vi "Or77200_DoXSteps.vi"(6 "MoveRef":refnum<vi>, 7 "Stop Ref":refnum<vi>, 8 "error In":errorcluster caption="error out", 9 "Dir (Dec:F)":bool caption="Dir", 10 "Steps":u32, 11 "Port":refnum<visa-resource-name>) -> (0 "sortie d'erreur":errorcluster, 2 "sortie 1":i32, 3 "Port Out":refnum<visa-resource-name>)   [LabVIEW 2019]
uses:
  <userlib>/GenProg/WritebyWeakRefBool.vi
  <userlib>/GenProg/ReadbyWeakRefBool.vi
panel:
  out "Moving":bool
  in  "Stop":bool
  out "Response":string
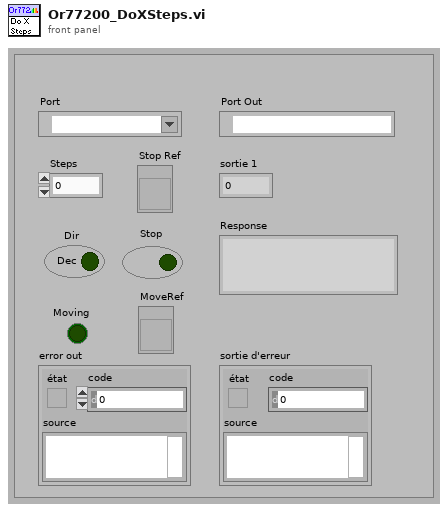
[diagram p1: front panel]
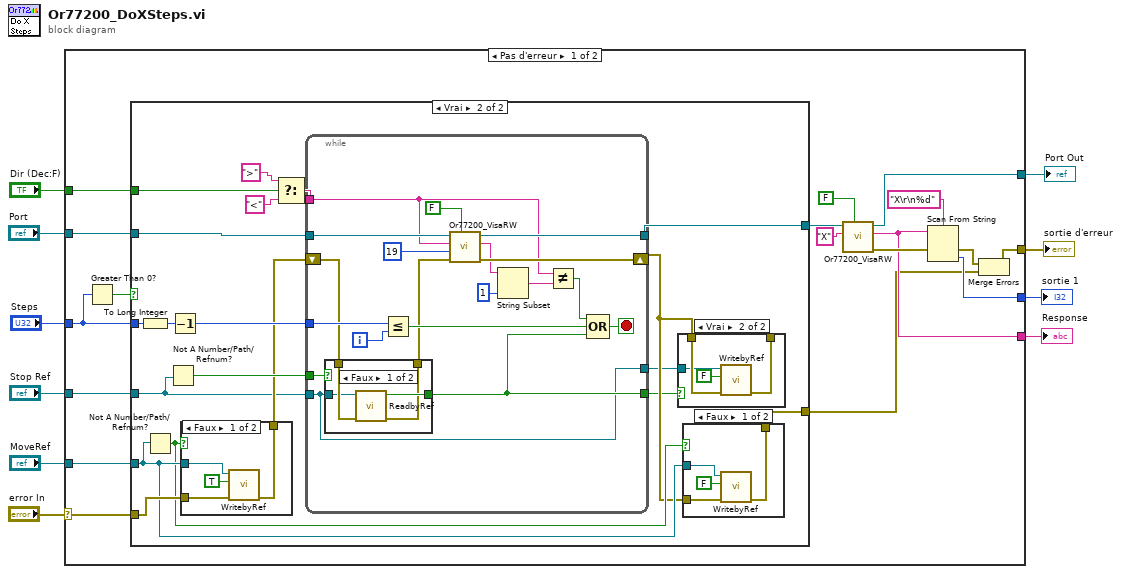
[diagram p0: block diagram]
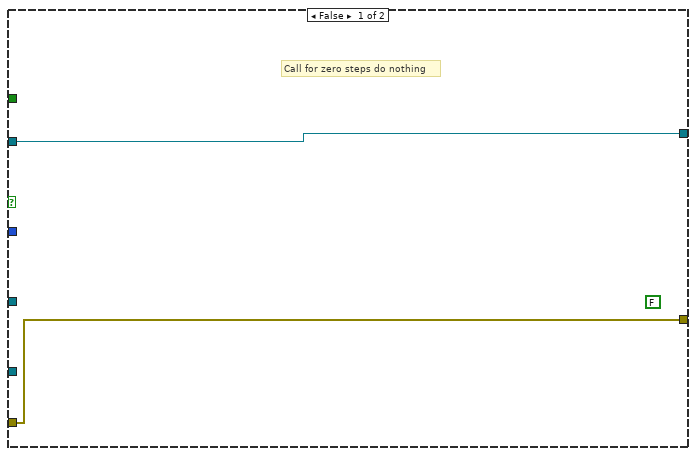
[diagram p2: hidden frame]
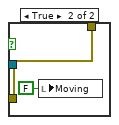
[diagram p4: hidden frame]
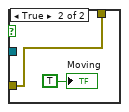
[diagram p5: hidden frame]
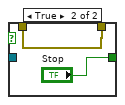
[diagram p6: hidden frame]
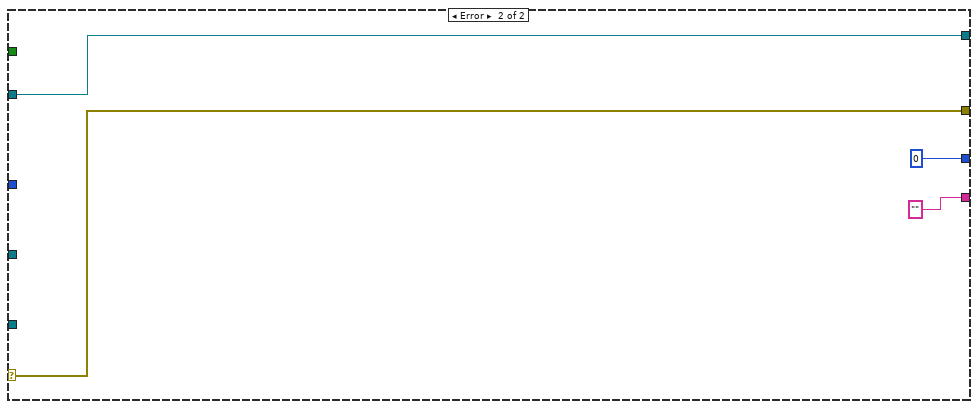
[diagram p7: hidden frame]
diagram:
  n1 = case shown="Pas d'erreur" "error In" {
    selector: "error In" -> [w18 w94]
    tunnel: "Port" -> [w28 w95]
    tunnel: "Dir (Dec:F)" -> [w27 _]
    tunnel: "Steps" -> [w16 _]
    tunnel: [w23 0] -> w7
    tunnel: [w14 w94] -> w6
    tunnel: [w21 w95] -> w5
    tunnel: "Stop Ref" -> [w19 _]
    tunnel: [w20 "" ("Response")] -> w3
    tunnel: "MoveRef" -> [w11 _]
    frame No Error {
      n2 = Greater Than 0?(x=w16) -> (x > 0?=w17:bool)
      n3 = case shown="Vrai" w17 {
        tunnel: w28 -> [w29 w49]
        tunnel: w27 -> [_ w48]
        tunnel: w16 -> [_ w47]
        tunnel: [w30 w37] -> w13
        tunnel: [w29 w45] -> w25
        tunnel: w19 -> [_ w34]
        tunnel: w18 -> [w30 w39]
        tunnel: w11 -> [_ w36]
        frame False {
          (unwired) FALSE ("Stop")
          # "Call for zero steps do nothing"
        }
        frame True {
          n4 = To Long Integer(number=w47) -> (32bit integer=w41:i32)
          n5 = Not A Number/Path/Refnum?(number/path/refnum=w36) -> (NaN/Path/Refnum?=w35:bool)
          n6 = Not A Number/Path/Refnum?(number/path/refnum=w34) -> (NaN/Path/Refnum?=w42:bool)
          n7 = Decrement(x=w41) -> (x-1=w46:i32)
          n8 = case shown="Faux" w35 {
            tunnel: [w64 w66] -> w38
            tunnel: w36 -> [w63 _]
            tunnel: w39 -> [w62 w66]
            frame False {
              n9 = call-poly <userlib>:"WritebyRef.vi"("error in"=w62, "Valeur"=TRUE, "Control Ref"=w63) -> ("error out"=w64:errorcluster)  [unwired: 8 in]
            }
            frame True {
              "Moving" <- TRUE ("Moving")
            }
          }
          n10 = Select(t=">" ("Commande"), s=w48, f="<" ("Commande")) -> (s? t:f=w43:string)
          n11 = while {
            tunnel: w49 -> [w85]
            shift-right: [w84] -> w33
            shift-left: w38 -> [w75]
            tunnel: w43 -> [w78]
            tunnel: w46 -> [w82]
            tunnel: [w81] -> w45
            tunnel: w42 -> [w73]
            tunnel: w34 -> [w67]
            tunnel: [w68] -> w32
            tunnel: [w67] -> w31
            i -> [w83]
            stop <- w77 stop-if-true
            n12 = case shown="Faux" w73 {
              tunnel: [w89 "Stop"] -> w68
              tunnel: w75 -> [w88 w90]
              tunnel: [w87 w90] -> w74
              tunnel: w67 -> [w86 _]
              frame False {
                n13 = call-poly <userlib>:"ReadbyRef.vi"("error in"=w88, "Control Ref"=w86) -> ("error out"=w87:errorcluster, "Valeur"=w89:bool)  [unwired: 8 in]
              }
              frame True {
              }
            }
            n14 = Less Or Equal?(x=w82, y=w83) -> (x <= y?=w76:bool)
            n15 = call <userlib>:"Or77200_VisaRW.vi"("Use LF-Cr"=FALSE, "error in"=w74, "ByteToRd"=u32 19, "Commande"=w78, "Port"=w85) -> ("error out"=w84:errorcluster, "Response"=w72:string, "Port Out"=w81:refnum<visa-resource-name>)  [unwired: 3 in, 1 out]
            n16 = String Subset(string=w72, length (rest)=1 ("longueur (reste)")) -> (substring=w79:string)  [unwired: 1 in]
            n17 = Not Equal?(x=w78, y=w79) -> (x != y?=w71:bool)
            n18 = Compound Arithmetic op=OR(w71, w76, w68) -> (w77:bool)
          }
          n19 = case shown="Vrai" w32 {
            tunnel: w33 -> [w50 w54]
            tunnel: [w50 w53] -> _
            tunnel: w31 -> [_ w52]
            frame False {
            }
            frame True {
              n20 = call-poly <userlib>:"WritebyRef.vi"("error in"=w54, "Valeur"=FALSE, "Control Ref"=w52) -> ("error out"=w53:errorcluster)  [unwired: 8 in]
            }
          }
          n21 = case shown="Faux" w35 {
            tunnel: [w58 w60] -> w37
            tunnel: w36 -> [w57 _]
            tunnel: w33 -> [w56 w60]
            frame False {
              n22 = call-poly <userlib>:"WritebyRef.vi"("error in"=w56, "Valeur"=FALSE, "Control Ref"=w57) -> ("error out"=w58:errorcluster)  [unwired: 8 in]
            }
            frame True {
              n23 = local write "Moving"(FALSE ("Moving")) -> ()
            }
          }
        }
      }
      n24 = call <userlib>:"Or77200_VisaRW.vi"("Use LF-Cr"=FALSE, "Commande"="X", "Port"=w25) -> ("error out"=w22:errorcluster, "Response"=w20:string, "Port Out"=w21:refnum<visa-resource-name>)  [unwired: 5 in, 1 out]
      n25 = Scan From String(format string="X\r\n%d" ("chaîne de format"), input string=w20, error in=w22) -> (error out=w15:errorcluster, output 1=w23:i32)  [unwired: 2 in, 2 out]
      n26 = Merge Errors(w15, w13) -> (w14:errorcluster)
    }
    frame Error {
    }
  }
  "sortie d'erreur" <- w6
  "sortie 1" <- w7
  "Port Out" <- w5
  "Response" <- w3
